vi "Messung.vi"(6 "Faktor2 (1)":dbl=1.0, 7 "Timeout (10000 ms)":u32=10000, 8 "error in":errorcluster, 9 "Points (6000)":i32=6000, 10 "Source Channel (0: Channel 1)":i32(ring) items=["Channel 1"=0, "Channel 2"=1, "Channel 3"=2, "Channel 4"=3, "Waveform Memory 1"=5, "Waveform Memory 2"=6, "Serial Bus 1"=7, "Serial Bus 2"=8, "Digital Bus Low"=9, "Digital Bus High "=10, "Digital Bus 1"=11, "Digital Bus 2"=12, "Function 1"=32, "Function 2"=33, "Function 3"=34, "Function 4"=35, "Math 1"=36, "Math 2"=37, "Math 3"=38, "Math 4"=39], 11 "VISA resource name(OZ)":refnum<visa-resource-name>="USB0::0x0957::0x179B::MY54313507::INSTR") -> (0 "error out":errorcluster, 1 "Messdaten":dbl[](array[numeric]), 2 "Waveform Data":waveform(dbl)(graph), 3 "VISA resource name out":refnum<visa-resource-name>)   [LabVIEW 2016]
doc: "Nimmt die auf den Oszilloskop angezeigte Kurve auf. Anschliesend wird bei den Messdaten noch der Offset des Oszilloskop abgezogen."
uses:
  <instrlib>/Agilent 2000 3000 X-Series/Agilent 2000 3000 X-Series.lvlib
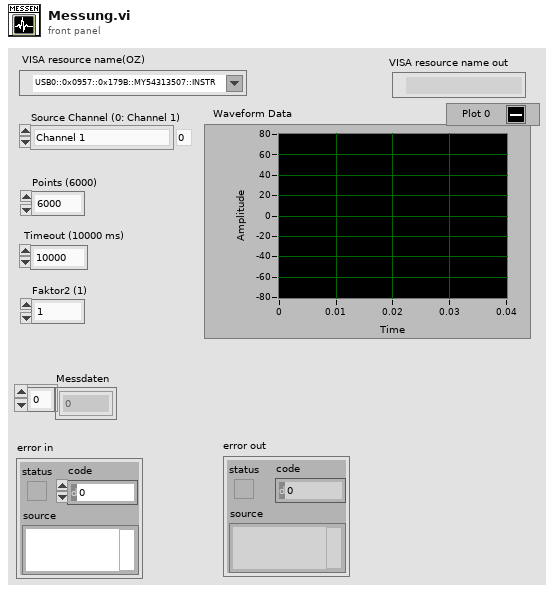
[diagram p1: front panel]
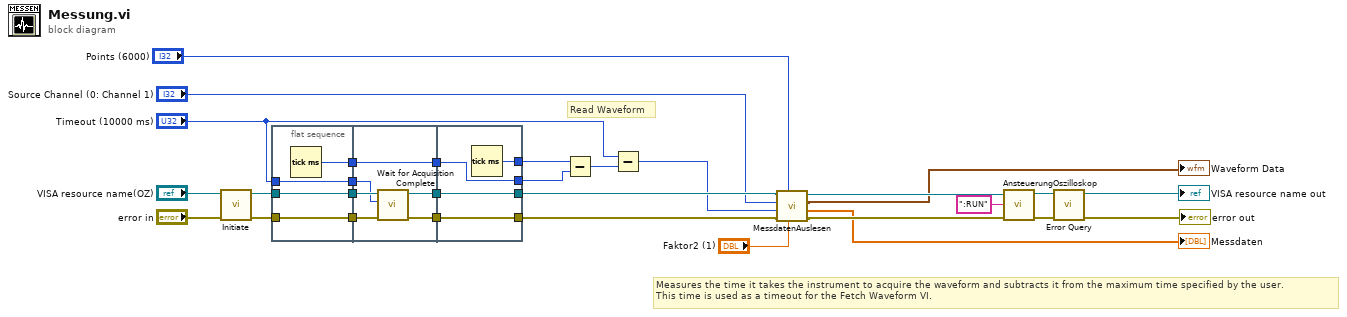
[diagram p0: block diagram]
diagram:
  # "Measures the time it takes the instrument to acquire the waveform and subtracts it from the maximum time specified by the user.\nThis time is used as a timeout for the Fetch Waveform VI."
  # "Read Waveform"
  n1 = call <instrlib>:"Initiate.vi"("error in (no error)"="error in", "VISA resource name"="VISA resource name(OZ)") -> ("error out"=w18:errorcluster, "VISA resource name out"=w19:refnum<visa-resource-name>)  [unwired: 8 in]
  n2 = flat-sequence {
    tunnel: w19 -> [w33]
    tunnel: [w33] -> w30
    tunnel: w18 -> [w32]
    tunnel: [w32] -> w29
    tunnel: "Timeout (10000 ms)" -> [w31]
    tunnel: [w31] -> w28
    tunnel: [w34] -> w27
    tunnel: w30 -> [w40]
    tunnel: [w38] -> w26
    tunnel: w29 -> [w39]
    tunnel: [w37] -> w25
    tunnel: w28 -> [w36]
    tunnel: w27 -> [w35]
    tunnel: [w35] -> w24
    tunnel: [w43] -> w8
    tunnel: w26 -> [w43]
    tunnel: [w42] -> w10
    tunnel: w25 -> [w42]
    tunnel: [w41] -> w23
    tunnel: w24 -> [w41]
    tunnel: [w44] -> w22
    frame #0 {
      n3 = Tick Count (ms)() -> (millisecond timer value=w34:u32)
    }
    frame #1 {
      n4 = call <instrlib>:"Wait for Acquisition Complete.vi"("error in (no error)"=w39, "Maximum Time (10000)"=w36, "VISA resource name"=w40) -> ("error out"=w37:errorcluster, "VISA resource name out"=w38:refnum<visa-resource-name>)  [unwired: 7 in]
    }
    frame #2 {
      n5 = Tick Count (ms)() -> (millisecond timer value=w44:u32)
    }
  }
  n6 = Subtract(x=w22, y=w23) -> (x-y=w14:u32)
  n7 = Subtract(x="Timeout (10000 ms)", y=w14) -> (x-y=w2:u32)
  n8 = call "MessdatenAuslesen.vi"("Faktor2 (1)"="Faktor2 (1)", "Points"="Points (6000)", "error in"=w10, "Timeout (10000)"=w2, "Source Channel (0: Channel 1)"="Source Channel (0: Channel 1)", "VISA Name OZ in(OZ)"=w8) -> ("error out"=w9:errorcluster, "Messdaten"=→"Messdaten":dbl[], "Waveform Data"=→"Waveform Data":waveform(dbl), "VISA resource name out"=w7:refnum<visa-resource-name>)  [unwired: 2 in]
  n9 = call "AnsteuerungOszilloskop.vi"("Error_in"=w9, "Eingangs-String"=":RUN", "VISA Name OZ in(OZ)"=w7) -> ("Error_out"=w12:errorcluster, "VISA Name OZ out"=w13:refnum<visa-resource-name>)  [unwired: 6 in, 1 out]
  n10 = call <instrlib>:"Error Query.vi"("error in (no error)"=w12, "VISA resource name"=w13) -> ("error out"=→"error out":errorcluster, "VISA resource name out"=→"VISA resource name out":refnum<visa-resource-name>)  [unwired: 6 in, 2 out]
